vi "Read Typedef Description (variant).vi"(8 "error in (no error)":errorcluster, 9 "variant in":variant) -> (0 "error out":errorcluster, 1 "variant out":variant, 2 "VI description":string)   [LabVIEW 2019, in "JSON-Schema.lvlib"]
doc: "Reads the <b>VI description</b> from a typedef wired to <b>variant in</b>"
uses:
  JSON-Schema.lvlib
  <vilib>/Utility/Data Type/NI_Data Type.lvlib
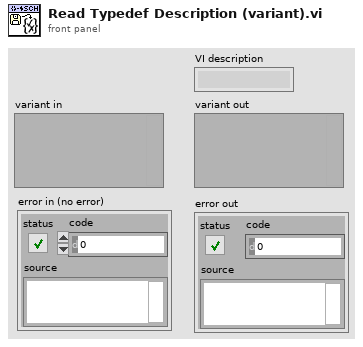
[diagram p1: front panel]
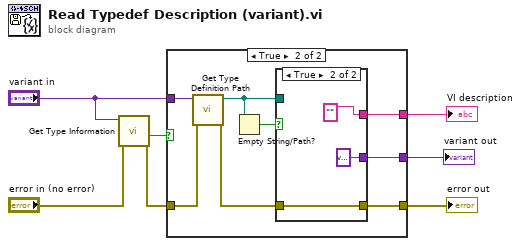
[diagram p0: block diagram]
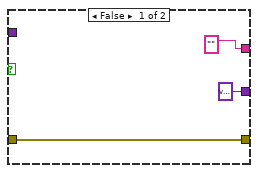
[diagram p2: hidden frame]
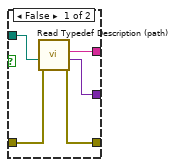
[diagram p3: hidden frame]
diagram:
  n1 = call <vilib>:"Get Type Information.vi"("error in (no error)"="error in (no error)", "variant"="variant in") -> ("error out"=w3:errorcluster, "type definition"=w2:bool)  [unwired: 5 in, 3 out]
  n2 = case shown="True" w2 {
    tunnel: [w9 w14] -> w7
    tunnel: ["" ("VI Description") w18] -> w6
    tunnel: "variant in" -> [_ w16]
    tunnel: w3 -> [w9 w15]
    tunnel: [variant ("Value") w11] -> w1
    frame False {
    }
    frame True {
      n3 = call <vilib>:"Get Type Definition Path.vi"("error in (no error)"=w15, "variant"=w16) -> ("error out"=w17:errorcluster, "type definition path"=w12:path)  [unwired: 8 in]
      n4 = Empty String/Path?(string/path=w12) -> (empty?=w13:bool)
      n5 = case shown="True" w13 {
        tunnel: [w21 "" ("VI Description")] -> w18
        tunnel: w17 -> [w23 w26]
        tunnel: w12 -> [w20 _]
        tunnel: [w22 w26] -> w14
        tunnel: [w19 variant ("Value")] -> w11
        frame False {
          n6 = call "Read Typedef Description (path).vi"("error in (no error)"=w23, "ctl path"=w20) -> ("error out"=w22:errorcluster, "variant out"=w19:variant, "VI description"=w21:string)  [unwired: 7 in]
        }
        frame True {
        }
      }
    }
  }
  "error out" <- w7
  "VI description" <- w6
  "variant out" <- w1
